vi "WriteCalibrationFile.vi"(8 "error in (no error)":errorcluster, 10 "CalibrationState":T1, 11 "Path":path) -> (0 "error out":errorcluster)   [LabVIEW 2012]
panel:
  # "CalibrationDone"
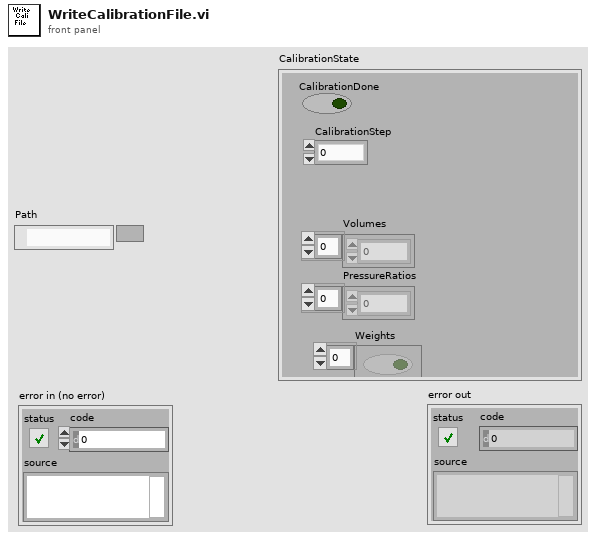
[diagram p1: front panel]
types:
  T1 = cluster{bool, "CalibrationStep":u32, "Volumes":dbl[], "PressureRatios":dbl[], "Weights":bool[]}
  T2 = enum16{"open", "replace", "create", "open or create", "replace or create", "replace or create with confirmation"}
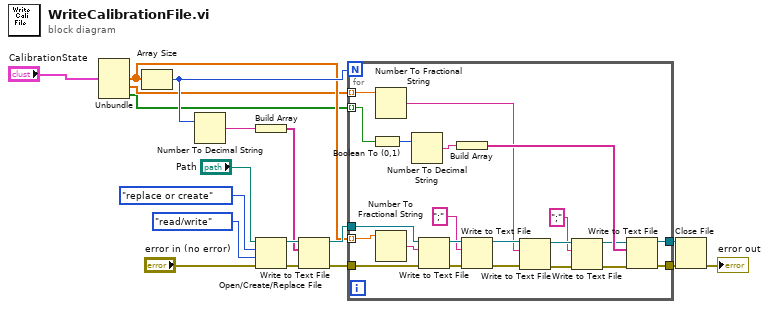
[diagram p0: block diagram]
diagram:
  n1 = Unbundle("CalibrationState") -> ("Volumes"=w5:dbl[], "PressureRatios"=w4:dbl[], "Weights"=w1:bool[])  [unwired: 2 out]
  n2 = Array Size(array=w5) -> (size(s)=w8:i32)
  n3 = Number To Decimal String(number=w8) -> (decimal integer string=w3:string)  [unwired: 1 in]
  n4 = Build Array(w3) -> (w2:string[])
  n5 = Open/Create/Replace File(file path (use dialog)="Path", error in="error in (no error)", operation (0:open)=T2."replace or create", access (0:read/write)=enum16{"read/write", "read-only", "write-only"}."read/write") -> (refnum out=w13:refnum<file>, error out=w12:errorcluster)  [unwired: 2 in, 1 out]
  n6 = Write to Text File(file (use dialog)=w13, text=w2, error in=w12) -> (refnum out=w6:refnum<file>, error out=w9:errorcluster)  [unwired: 1 in, 1 out]
  n7 = for {
    N: w8 -> [_]
    tunnel: [w40] -> w10
    tunnel: w9 -> [w39]
    tunnel: [w36] -> w7
    tunnel: w6 -> [w35]
    tunnel: w5 -> [w34] mode=indexing
    tunnel: w4 -> [w33] mode=indexing
    tunnel: w1 -> [w27] mode=indexing
    n8 = Boolean To (0,1)(Boolean=w27) -> (0, 1=w26:i16)
    n9 = Number To Fractional String(number=w33) -> (F-format string=w24:string)  [unwired: 3 in]
    n10 = Number To Fractional String(number=w34) -> (F-format string=w31:string)  [unwired: 3 in]
    n11 = Number To Decimal String(number=w26) -> (decimal integer string=w25:string)  [unwired: 1 in]
    n12 = Write to Text File(file (use dialog)=w35, text=w31, error in=w39) -> (refnum out=w37:refnum<file>, error out=w38:errorcluster)  [unwired: 1 in, 1 out]
    n13 = Build Array(w25) -> (w32:string[])
    n14 = Write to Text File(file (use dialog)=w37, text=";", error in=w38) -> (refnum out=w29:refnum<file>, error out=w28:errorcluster)  [unwired: 1 in, 1 out]
    n15 = Write to Text File(file (use dialog)=w29, text=w24, error in=w28) -> (refnum out=w22:refnum<file>, error out=w23:errorcluster)  [unwired: 1 in, 1 out]
    n16 = Write to Text File(file (use dialog)=w22, text=";", error in=w23) -> (refnum out=w21:refnum<file>, error out=w20:errorcluster)  [unwired: 1 in, 1 out]
    n17 = Write to Text File(file (use dialog)=w21, text=w32, error in=w20) -> (refnum out=w36:refnum<file>, error out=w40:errorcluster)  [unwired: 1 in, 1 out]
  }
  n18 = Close File(refnum=w7, error in=w10) -> (error out=→"error out":errorcluster)  [unwired: 1 out]
